vi "RTS Read Wago Configuration.vi"(8 "Error In":errorcluster, 9 "RTS Config Setup Output in":T1, 11 "Search File Path in":path) -> (0 "error out":errorcluster, 1 "RTS Config Setup Output out":T1, 3 "Search File Path Output":path)   [LabVIEW 2016]
uses:
  Type Definitions/RTS Configuration Setup.ctl
  Type Definitions/RTS Wago Config.ctl
  Type Definitions/RTS APLUS Config.ctl
  Type Definitions/RTS Yokogawa MX Config.ctl
  Type Definitions/RTS Replay Server Control.ctl
  Type Definitions/RTS Server Configuration.ctl
  Type Definitions/RTS Station Settions TCP Comms.ctl
  Type Definitions/RTS Chamber Save Status.ctl
  Type Definitions/RTS Test Pattern.ctl
  <vilib>/Utility/file.llb/Read Delimited Spreadsheet (string).vi
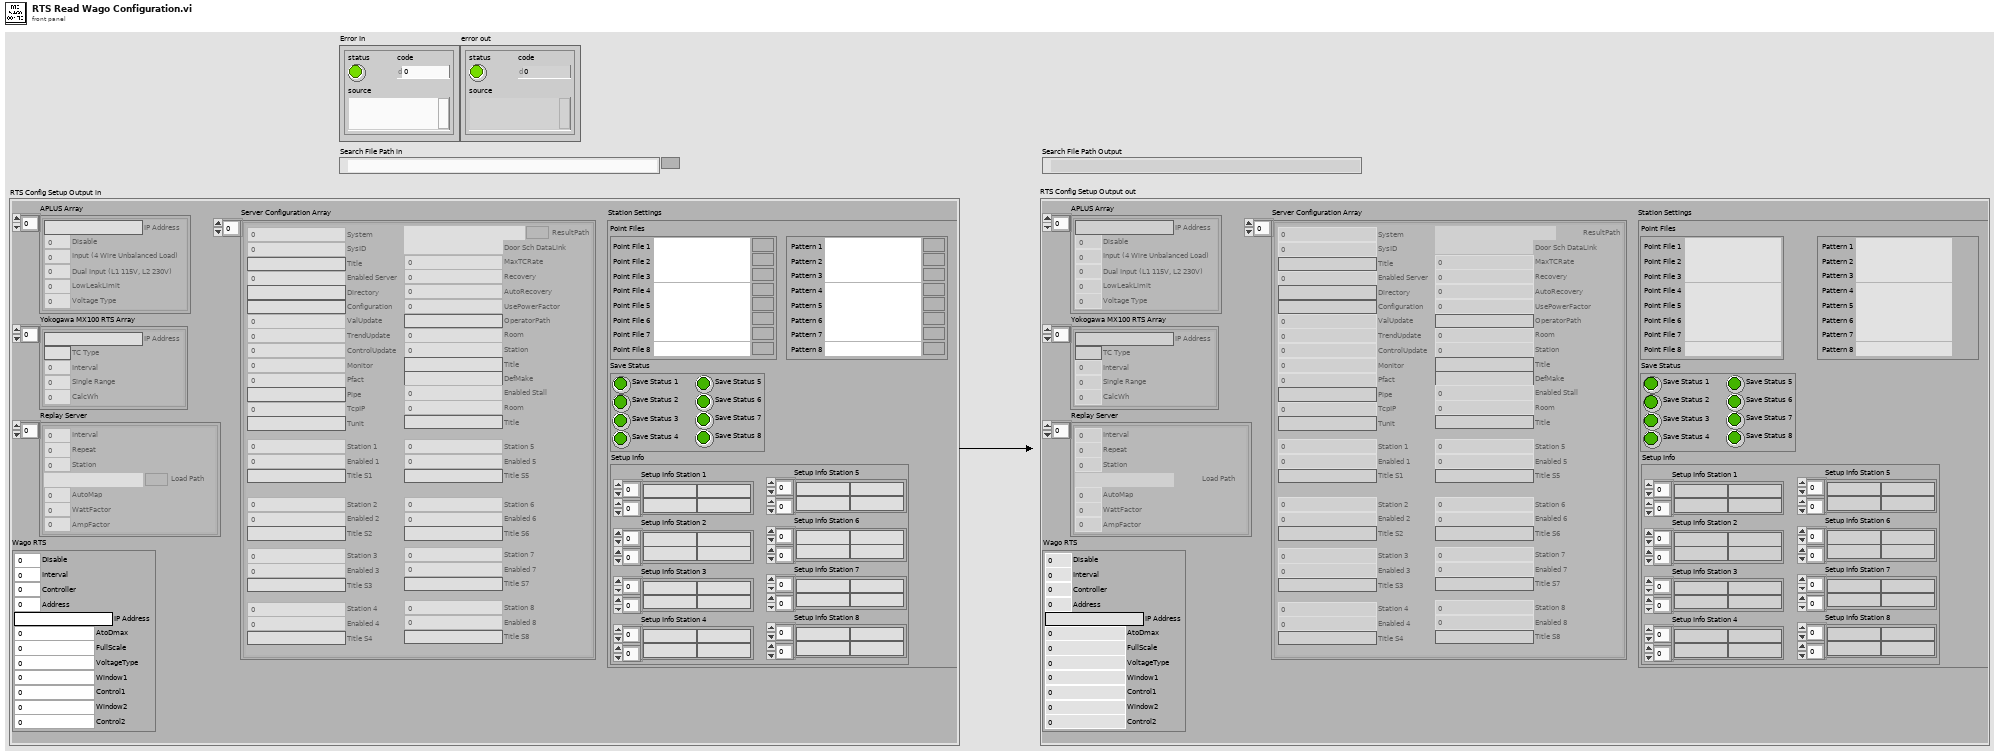
[diagram p1: front panel]
types:
  T1 = typedef "RTS Configuration Setup.ctl" = cluster{"Wago RTS":T2, "APLUS Array":T3[], "Yokogawa MX100 RTS Array":T4[], "Replay Server":T5[], "Server Configuration Array":T6[], "Station Settings":T7}
  T2 = typedef "RTS Wago Config.ctl" = cluster{"Disable":u16, "Interval":u16, "Controller":u16, "Address":u16, "IP Address":string, "AtoDmax":u16, "FullScale":u16, "VoltageType":u16, "Window1":u16, "Control1":u16, "Window2":u16, "Control2":u16}
  T3 = typedef "RTS APLUS Config.ctl" = cluster{"Disable":u16, "IP Address":string, "Input (4 Wire Unbalanced Load)":u16, "Dual Input (L1 115V, L2 230V)":u16, "LowLeakLimit":dbl, "Voltage Type":u16}
  T4 = typedef "RTS Yokogawa MX Config.ctl" = cluster{"IP Address":string, "TC Type":string, "Interval":u16, "Single Range":u16, "CalcWh":u16}
  T5 = typedef "RTS Replay Server Control.ctl" = cluster{"Interval":i16, "Repeat":u16, "Station":u16, "Load Path":path, "AutoMap":u16, "WattFactor":dbl, "AmpFactor":dbl}
  T6 = typedef "RTS Server Configuration.ctl" = cluster{"System":u16, "SysID":u16, "Title":string, "Enabled Server":u16, "Directory":string, "Configuration":string, "ValUpdate":u16, "TrendUpdate":u16, "ControlUpdate":u16, "Monitor":u16, "Pfact":u16, "Pipe":string, "TcpIP":u16, "Tunit":string, "ResultPath":path, "Door Sch DataLink":path, "MaxTCRate":u16, "Recovery":u16, "AutoRecovery":u16, "UsePowerFactor":u16, "OperatorPath":string, "Room":u16, "Station":u16, "Title":string, "DefMake":string, "Enabled Stall":u16, "Room":u16, "Title":string, "Station 1":u16, "Enabled 1":u16, "Station 2":u16, "Enabled 2":u16, "Station 3":u16, "Enabled 3":u16, "Station 4":u16, "Enabled 4":u16, "Station 5":u16, "Enabled 5":u16, "Station 6":u16, "Enabled 6":u16, "Station 7":u16, "Enabled 7":u16, "Station 8":u16, "Enabled 8":u16, "Title S1":string, "Title S2":string, "Title S3":string, "Title S5":string, "Title S6":string, "Title S7":string, "Title S8":string, "Title S4":string}
  T7 = typedef "RTS Station Settions TCP Comms.ctl" = cluster{"Point Files":cluster{"Point File 1":path, "Point File 2":path, "Point File 3":path, "Point File 4":path, "Point File 5":path, "Point File 6":path, "Point File 7":path, "Point File 8":path}, "Save Status":T8, "Setup Info":cluster{"Setup Info Station 1":string[][], "Setup Info Station 2":string[][], "Setup Info Station 3":string[][], "Setup Info Station 4":string[][], "Setup Info Station 5":string[][], "Setup Info Station 6":string[][], "Setup Info Station 7":string[][], "Setup Info Station 8":string[][]}, "Chamber Test Pattern":T9}
  T8 = typedef "RTS Chamber Save Status.ctl" = cluster{"Save Status 1":bool, "Save Status 2":bool, "Save Status 3":bool, "Save Status 4":bool, "Save Status 5":bool, "Save Status 6":bool, "Save Status 7":bool, "Save Status 8":bool}
  T9 = typedef "RTS Test Pattern.ctl" = cluster{" Pattern 1":path, "Pattern 2":path, "Pattern 3":path, "Pattern 4":path, "Pattern 5":path, "Pattern 6":path, "Pattern 7":path, "Pattern 8":path}
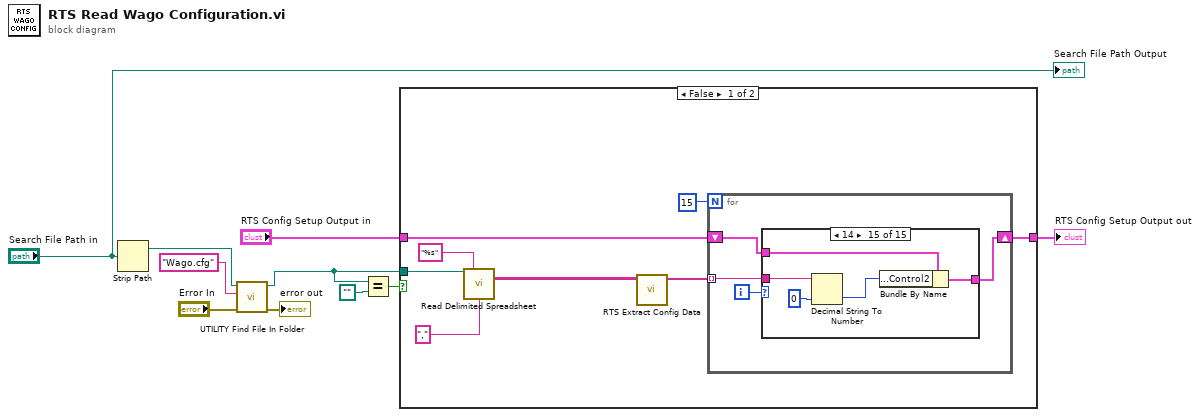
[diagram p0: block diagram]
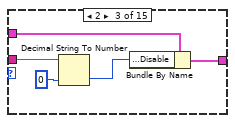
[diagram p4: hidden frame]
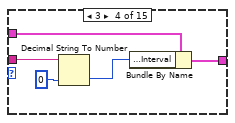
[diagram p5: hidden frame]
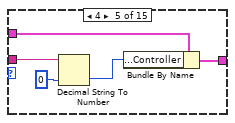
[diagram p6: hidden frame]
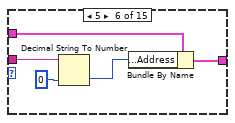
[diagram p7: hidden frame]
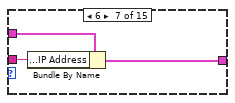
[diagram p8: hidden frame]
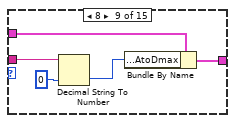
[diagram p10: hidden frame]
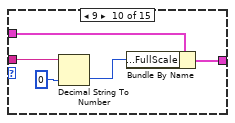
[diagram p11: hidden frame]
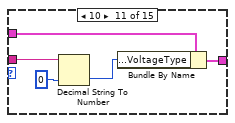
[diagram p12: hidden frame]
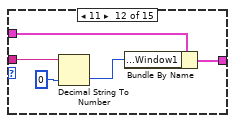
[diagram p13: hidden frame]
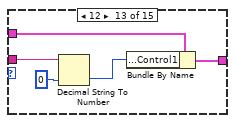
[diagram p14: hidden frame]
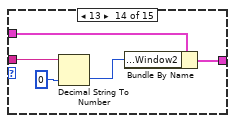
[diagram p15: hidden frame]
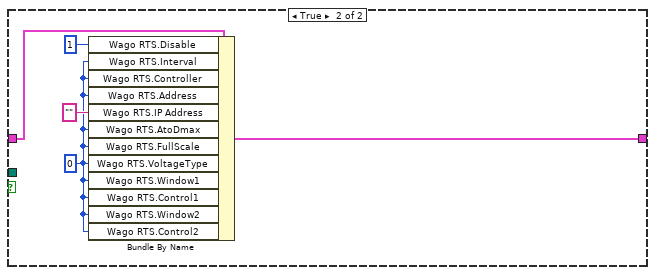
[diagram p16: hidden frame]
diagram:
  n1 = Strip Path(path="Search File Path in") -> (stripped path=w6:path)  [unwired: 1 out]
  n2 = call "UTILITY Find File In Folder.vi"("Error In"="Error In", "File Name"="Wago.cfg", "Path"=w6) -> ("Error Out"=→"error out":errorcluster, "appended path"=w3:path)  [unwired: 7 in]
  n3 = Equal?(x=w3, y=path "") -> (x = y?=w1:bool)
  n4 = case shown="False" w1 {
    tunnel: "RTS Config Setup Output in" -> [w14 w88]
    tunnel: [w13 w87] -> w4
    tunnel: w3 -> [w11 _]
    frame False {
      n5 = call-poly <vilib>:"Read Delimited Spreadsheet.vi"("file path (dialog if empty)"=w11, "format (%s)"="%s", "delimiter (\\t)"="," ("delimiter (\\t)")) -> ("all rows"=w16:string[][])  [unwired: 7 in, 5 out]
      n6 = call "RTS Extract Config Data.vi"("all rows"=w16) -> ("Array"=w15:string[])  [unwired: 9 in, 1 out]
      n7 = for {
        N: 15 -> [_]
        tunnel: w15 -> [w20] mode=indexing
        shift-right: [w19] -> w13
        shift-left: w14 -> [w21]
        i -> [w22]
        n8 = case shown="14" w22 {
          tunnel: w21 -> [w23 w24 w29 w32 w37 w41 w46 w48 w50 w55 w60 w65 w70 w75 w80]
          tunnel: w20 -> [_ _ w27 w30 w35 w40 w45 _ w49 w54 w59 w64 w69 w74 w79]
          tunnel: [w23 w24 w25 w31 w36 w42 w47 w48 w51 w56 w61 w66 w71 w76 w81] -> w19
          frame 0, Default {
          }
          frame 1 {
          }
          frame 2 {
            n9 = Decimal String To Number(string=w27, default (0L)=u16 0 ("default (0 I32)")) -> (number=w26:u16)  [unwired: 1 in, 1 out]
            n10 = Bundle By Name(cluster=w29, "Wago RTS.Disable"=w26) -> (w25:T1)
          }
          frame 3 {
            n11 = Decimal String To Number(string=w30, default (0L)=u16 0 ("default (0 I32)")) -> (number=w33:u16)  [unwired: 1 in, 1 out]
            n12 = Bundle By Name(cluster=w32, "Wago RTS.Interval"=w33) -> (w31:T1)
          }
          frame 4 {
            n13 = Decimal String To Number(string=w35, default (0L)=u16 0 ("default (0 I32)")) -> (number=w38:u16)  [unwired: 1 in, 1 out]
            n14 = Bundle By Name(cluster=w37, "Wago RTS.Controller"=w38) -> (w36:T1)
          }
          frame 5 {
            n15 = Decimal String To Number(string=w40, default (0L)=u16 0 ("default (0 I32)")) -> (number=w43:u16)  [unwired: 1 in, 1 out]
            n16 = Bundle By Name(cluster=w41, "Wago RTS.Address"=w43) -> (w42:T1)
          }
          frame 6 {
            n17 = Bundle By Name(cluster=w46, "Wago RTS.IP Address"=w45) -> (w47:T1)
          }
          frame 7 {
          }
          frame 8 {
            n18 = Decimal String To Number(string=w49, default (0L)=u16 0 ("default (0 I32)")) -> (number=w52:u16)  [unwired: 1 in, 1 out]
            n19 = Bundle By Name(cluster=w50, "Wago RTS.AtoDmax"=w52) -> (w51:T1)
          }
          frame 9 {
            n20 = Decimal String To Number(string=w54, default (0L)=u16 0 ("default (0 I32)")) -> (number=w57:u16)  [unwired: 1 in, 1 out]
            n21 = Bundle By Name(cluster=w55, "Wago RTS.FullScale"=w57) -> (w56:T1)
          }
          frame 10 {
            n22 = Decimal String To Number(string=w59, default (0L)=u16 0 ("default (0 I32)")) -> (number=w62:u16)  [unwired: 1 in, 1 out]
            n23 = Bundle By Name(cluster=w60, "Wago RTS.VoltageType"=w62) -> (w61:T1)
          }
          frame 11 {
            n24 = Decimal String To Number(string=w64, default (0L)=u16 0 ("default (0 I32)")) -> (number=w67:u16)  [unwired: 1 in, 1 out]
            n25 = Bundle By Name(cluster=w65, "Wago RTS.Window1"=w67) -> (w66:T1)
          }
          frame 12 {
            n26 = Decimal String To Number(string=w69, default (0L)=u16 0 ("default (0 I32)")) -> (number=w72:u16)  [unwired: 1 in, 1 out]
            n27 = Bundle By Name(cluster=w70, "Wago RTS.Control1"=w72) -> (w71:T1)
          }
          frame 13 {
            n28 = Decimal String To Number(string=w74, default (0L)=u16 0 ("default (0 I32)")) -> (number=w77:u16)  [unwired: 1 in, 1 out]
            n29 = Bundle By Name(cluster=w75, "Wago RTS.Window2"=w77) -> (w76:T1)
          }
          frame 14 {
            n30 = Decimal String To Number(string=w79, default (0L)=u16 0 ("default (0 I32)")) -> (number=w82:u16)  [unwired: 1 in, 1 out]
            n31 = Bundle By Name(cluster=w80, "Wago RTS.Control2"=w82) -> (w81:T1)
          }
        }
      }
    }
    frame True {
      w84 = u16 0 ("Wago RTS.Interval")
      n32 = Bundle By Name(cluster=w88, "Wago RTS.Disable"=u16 1, "Wago RTS.Interval"=w84, "Wago RTS.Controller"=w84, "Wago RTS.Address"=w84, "Wago RTS.IP Address"="", "Wago RTS.AtoDmax"=w84, "Wago RTS.FullScale"=w84, "Wago RTS.VoltageType"=w84, "Wago RTS.Window1"=w84, "Wago RTS.Control1"=w84, "Wago RTS.Window2"=w84, "Wago RTS.Control2"=w84) -> (w87:T1)
    }
  }
  "RTS Config Setup Output out" <- w4
  "Search File Path Output" <- "Search File Path in"
